vi "Op-Save-Recall.vi"(0 "VISA resource name":refnum<visa-resource-name>, 1 "operation":bool, 5 "source/destination\n(disk file :0)":u16(ring) items=["disk file ->", "memory 1", "memory 2", "memory 3", "memory 4"], 7 "file name (\"SAVED\") (max 8 chars)\n(no extension allowed)":string="SAVED", 9 "data type (measurement setup:0)":u16(ring) items=["measurement setup", "stress setup", "measurement setup and result data"], 11 "error in (no error)":errorcluster) -> (4 "VISA resource name out":refnum<visa-resource-name>, 15 "error out":errorcluster)   [LabVIEW 2016, in "Agilent 415X Series.lvlib"]
doc: "This VI saves or recalls measurement, stress, and trace information to the instrument's disk drive or one of the four internal memory locations."
uses:
  Agilent 415X Series.lvlib
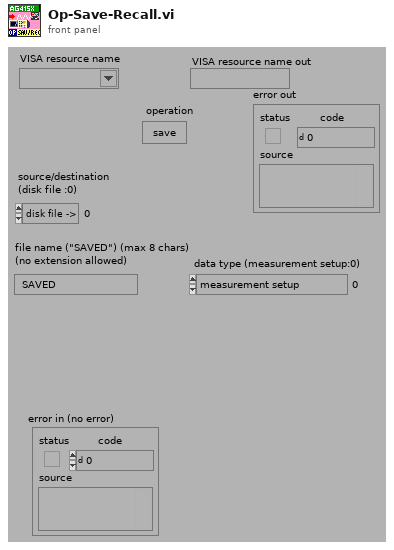
[diagram p1: front panel]
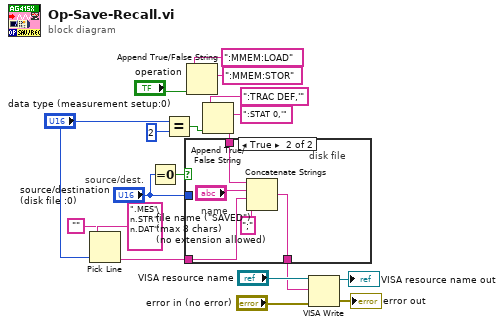
[diagram p0: block diagram]
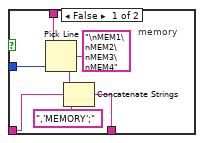
[diagram p2: hidden frame]
diagram:
  # "source/dest."
  n1 = Pick Line(string ("")="" ("Empty String Constant"), multi-line string=".MES'\n.STR'\n.DAT'", line index="data type (measurement setup:0)") -> (output string=w2:string)
  n2 = Equal To 0?(x="source/destination\n(disk file :0)") -> (x = 0?=w12:bool)
  n3 = Equal?(x="data type (measurement setup:0)", y=2) -> (x = y?=w15:bool)
  n4 = Append True/False String(1:"operation", 2:":MMEM:STOR", 3:":MMEM:LOAD") -> (0:w13:string)  [unwired: 1 in]
  n5 = Append True/False String(1:w15, 2:":STAT 0,'", 3:":TRAC DEF,'", 4:w13) -> (0:w11:string)
  n6 = case shown="True" w12 {
    tunnel: w11 -> [w27 w31]
    tunnel: "source/destination\n(disk file :0)" -> [w26 _]
    tunnel: [w23 w29] -> w6
    tunnel: w2 -> [w22 w30]
    frame False {
      # "memory"
      n7 = Pick Line(string ("")=w27, multi-line string="\nMEM1\nMEM2\nMEM3\nMEM4", line index=w26) -> (output string=w24:string)
      n8 = Concatenate Strings(w24, w22, ",'MEMORY';") -> (w23:string)
    }
    frame True {
      # "disk file"
      # "name"
      n9 = Concatenate Strings(w31, "file name (\"SAVED\") (max 8 chars)\n(no extension allowed)", w30, ";") -> (w29:string)
    }
  }
  n10 = VISA Write(VISA resource name="VISA resource name", write buffer=w6, error in (no error)="error in (no error)") -> (VISA resource name out=→"VISA resource name out":refnum<visa-resource-name>, error out=→"error out":errorcluster)  [unwired: 1 out]
